vi "DIM_DIO.reset.vi"(0 "i ref in":refnum<vi>, 3 "ms timeout (10000)":i32=10000, 5 "error in (no error)":errorcluster) -> (14 "i ref out":refnum<vi>, 17 "timed out":bool, 19 "error out":errorcluster)   [LabVIEW 2014, in "DIM_DIO.lvlib"]
doc: "Resets the output bit to FALSE.\n\nLicense Agreement for this software:\n\nCopyright (C)\nGesellschaft für Schwerionenforschung, GSI\nPlanckstr. 1\n64291 Darmstadt\nGermany\n\nContact: D.Beck@gsi.de \n\nThis program is free software; you can redistribute it and/or modify it under the terms of the GNU General Public License as published by the Free Software Foundation; either version 2 of the license, or (at your option) any later version.\n\nThis program is distributed in the hope that it will be useful, but WITHOUT ANY WARRANTY; without even the implied warranty of MERCHANTABILITY or FITNESS FOR A PARTICULAR PURPOSE. See the GNU General License for more details (http://www.gnu.org).\n\nGesellschaft für Schwerionenforschung, GSI\nPlanckstr. 1, 64291 Darmstadt, Germany\nFor all questions and ideas contact: M.Richter@gsi.de, H.Brand@gsi.de or D.Beck@gsi.de.\nLast update: 17-JUN-2004"
uses:
  DIM_DIO.lvlib
  CSCore/CSApplicationBaseClasses/DeviceBase/DeviceBase.lvlib
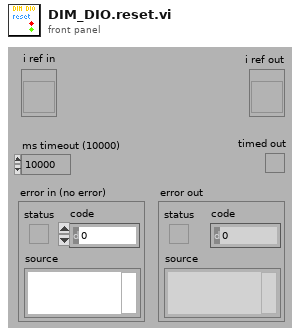
[diagram p1: front panel]
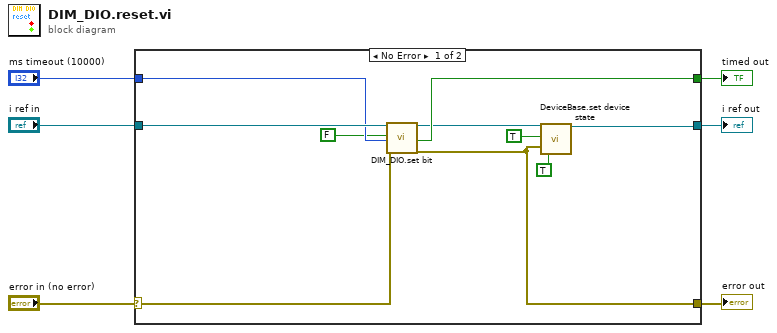
[diagram p0: block diagram]
diagram:
  n1 = case shown="No Error" "error in (no error)" {
    selector: "error in (no error)" -> [w13 w18]
    tunnel: [w10 w18] -> w5
    tunnel: "i ref in" -> [w16 w17]
    tunnel: [w9 w17] -> w3
    tunnel: "ms timeout (10000)" -> [w14 _]
    tunnel: [w15 _] -> w1
    frame No Error {
      n2 = call "DIM_DIO.set bit.vi"("i ref in"=w16, "bitValue"=FALSE, "ms timeout (10000)"=w14, "error in (no error)"=w13) -> ("i ref out"=w11:refnum<vi>, "timed out"=w15:bool, "error out"=w10:errorcluster)  [unwired: 13 in]
      n3 = call "DeviceBase.set device state.vi"("i ref in"=w11, "implicit"=TRUE, "device error"=w10, "mayResetError (FALSE)"=TRUE) -> ("i ref out"=w9:refnum<vi>)  [unwired: 13 in, 2 out]
    }
    frame Error {
    }
  }
  "error out" <- w5
  "i ref out" <- w3
  "timed out" <- w1
